vi "rad_Retrieve Image Wrapper.vi"(7 "Deployment Notifiers":T6, 8 "error in (no error)":errorcluster, 9 "AppImage Properties":T3, 10 "image file path":path, 11 "Target settings":T1={"Hostname"="", "Serial number"="", "Product name"="", "Product code"=0, "System status"="", "Credential type"=enum."None/Unlocked", "User added?"=FALSE, "Primary NIC"={"MAC address"="", "IP Address Request Mode"=2, "IP address"="", "Subnet mask"="", "Gateway"="", "DNS server"=""}} {"Primary NIC"."IP Address Request Mode" items=["Static"=1, "DHCP/Link-Local"=2, "Link-Local Only"=4, "DHCP Only"=8]}) -> (0 "error out":errorcluster, 3 "Canceled":bool)   [LabVIEW 2020]
uses:
  TypeDefs/rad_Deployment Progress Data Type.ctl
  TypeDefs/rad_Deployment Notifiers.ctl
  TypeDefs/rad_Deployment Status Data Type.ctl
  TypeDefs/rad_Application Image Properties.ctl
  TypeDefs/rad_FPGA Properties.ctl
  TypeDefs/rad_FPGA Flash Properties.ctl
  support/SubVIs/Target Information.ctl
  Targets/TypeDefs/rad_Target Network Settings.ctl
  <vilib>/nisyscfg/Software 1.2.ctl
  <vilib>/nisyscfg/Component Type.ctl
  <vilib>/nisyscfg/Create System Image (Folder).vi
  <vilib>/nisyscfg/Close (System).vi
  <vilib>/nisyscfg/nisyscfg.lvlib
panel:
  in  "Stop Checking for Events":bool
  out "Progress":T7 scale=0.0..100.0
  out "Status":string
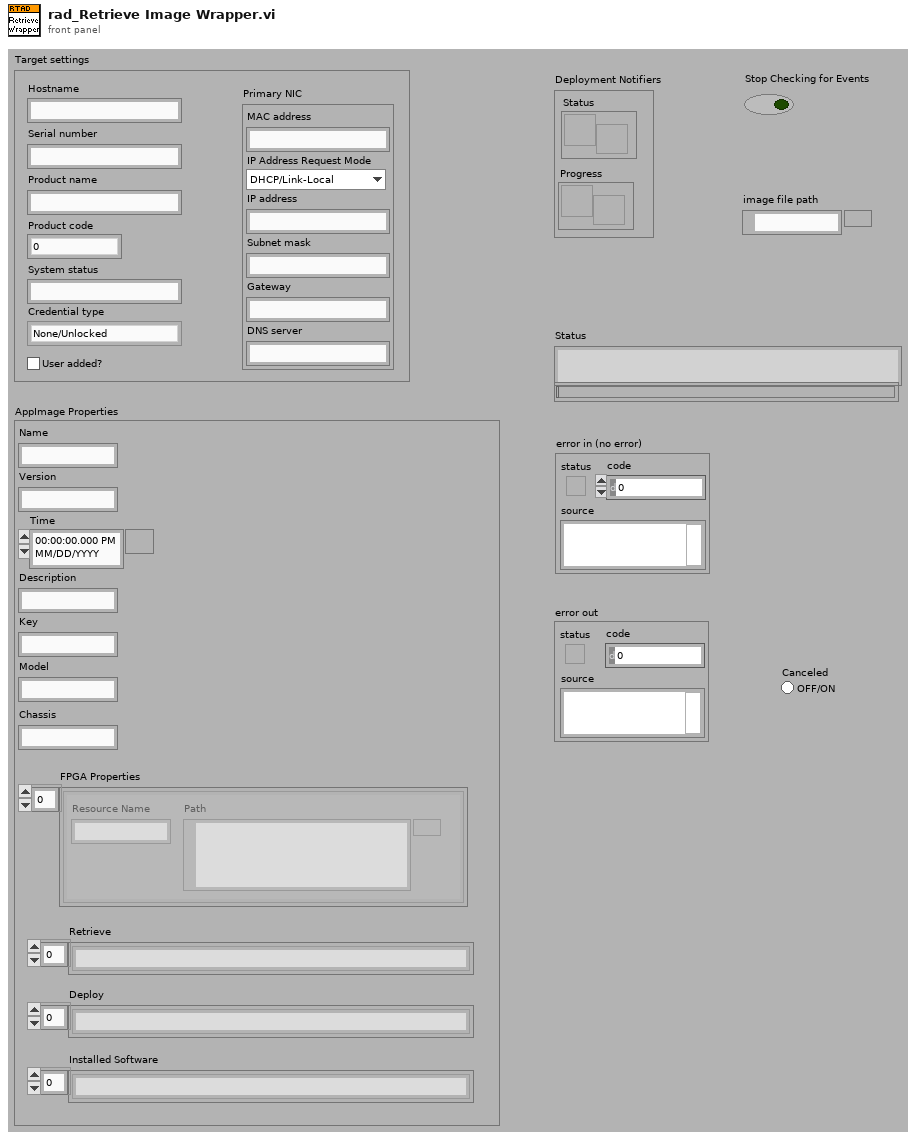
[diagram p1: front panel]
types:
  T1 = typedef "Target Information.ctl" = cluster{"Hostname":string, "Serial number":string, "Product name":string, "Product code":i32, "System status":string, "Credential type":enum16{"None/Unlocked", "FTP Password", "NIAuth Credentials"}, "User added?":bool, "Primary NIC":T2}
  T2 = typedef "rad_Target Network Settings.ctl" = cluster{"MAC address":string, "IP Address Request Mode":i32, "IP address":string, "Subnet mask":string, "Gateway":string, "DNS server":string}
  T3 = typedef "rad_Application Image Properties.ctl" = cluster{"Name":string, "Version":string, "Time":timestamp, "Description":string, "Key":string, "Chassis":string, "FPGA Properties":T4, "Model":string, "Retrieve":string[], "Deploy":string[], "Installed Software":string[]}
  T4 = typedef "rad_FPGA Properties.ctl" = T5[]
  T5 = typedef "rad_FPGA Flash Properties.ctl" = cluster{"Resource Name":string, "Path":path}
  T6 = typedef "rad_Deployment Notifiers.ctl" = cluster{"Status":refnum<notifier>, "Progress":refnum<notifier>}
  T7 = typedef "rad_Deployment Progress Data Type.ctl" = i8
  T8 = typedef "nisyscfg.lvlib/Software 1.2.ctl" = cluster{"title":string, "description":string, "ID":string, "version":string, "component type":T9}
  T9 = typedef "nisyscfg.lvlib/Component Type.ctl" = u32
  T10 = enum32{"state changed", "beginning restart", "getting file", "putting file", "creating directory", "deleting file", "deleting directory", "enumerating file system", "renaming file", "current component", "operation progress", "downloading file", "unpacking file", "running install script"}
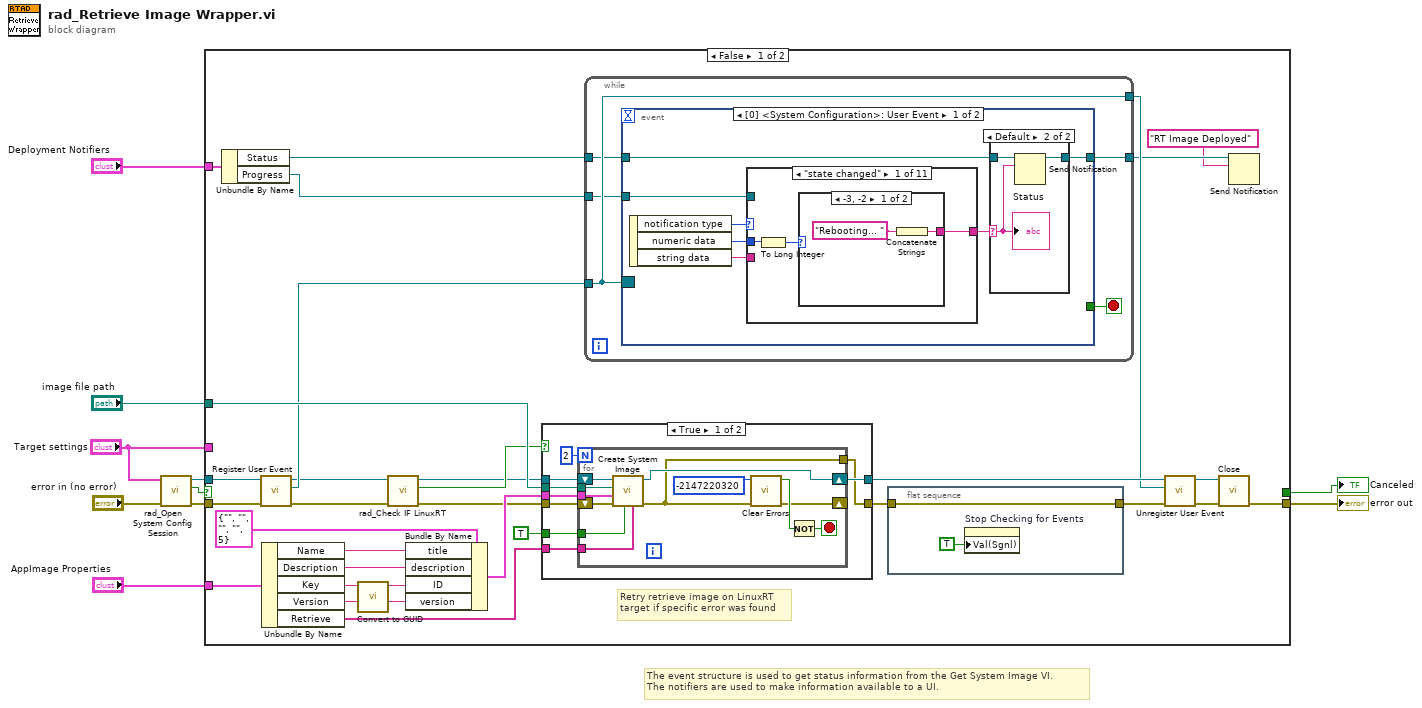
[diagram p0: block diagram]
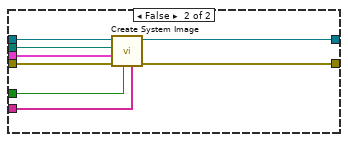
[diagram p2: hidden frame]
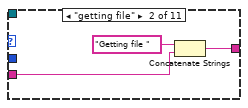
[diagram p5: hidden frame]
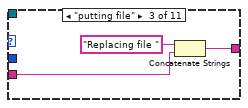
[diagram p6: hidden frame]
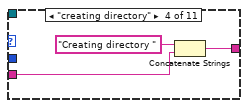
[diagram p7: hidden frame]
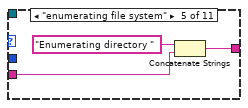
[diagram p8: hidden frame]
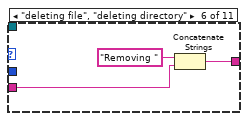
[diagram p9: hidden frame]
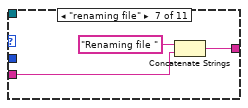
[diagram p10: hidden frame]
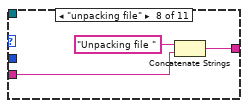
[diagram p11: hidden frame]
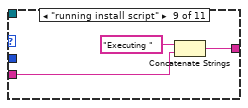
[diagram p12: hidden frame]
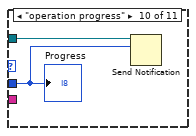
[diagram p13: hidden frame]
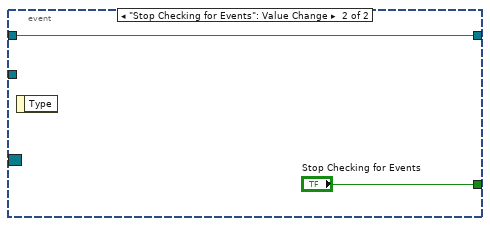
[diagram p15: hidden frame]
diagram:
  # "The event structure is used to get status information from the Get System Image VI. \nThe notifiers are used to make information available to a UI."
  n1 = call "rad_Open System Config Session.vi"("error in (no error)"="error in (no error)", "Target settings"="Target settings") -> ("error out"=w3:errorcluster, "Cancelled"=w2:bool, "Session out"=w4:refnum<k21>)  [unwired: 6 in, 1 out]
  n2 = case shown="False" w2 {
    selector: w2 -> [_ w122]
    tunnel: [w41 w123] -> w8
    tunnel: "image file path" -> [w40 _]
    tunnel: w4 -> [w39 _]
    tunnel: w3 -> [w38 w123]
    tunnel: "Deployment Notifiers" -> [w25 _]
    tunnel: "AppImage Properties" -> [w24 _]
    tunnel: [_ w122] -> w6
    tunnel: "Target settings" -> [_ _]
    frame False {
      # "Retry retrieve image on LinuxRT\ntarget if specific error was found"
      n3 = Unbundle By Name(w25) -> ("Status"=w27:refnum<notifier>, "Progress"=w26:refnum<notifier>)
      n4 = call <vilib>:"Register User Event.vi"("error in (no error)"=w38, "Session in"=w39) -> ("error out"=w14:errorcluster, "Event Registration out"=w37:refnum<event-registration>, "Session out"=w15:refnum<k21>)  [unwired: 7 in]
      n5 = Unbundle By Name(w24) -> ("Name"=w22:string, "Description"=w21:string, "Key"=w18:string, "Version"=w20:string, "Retrieve"=w16:string[])
      n6 = call "Convert to GUID.vi"("Key"=w18) -> ("GUID"=w17:string)  [unwired: 10 in]
      n7 = call "rad_Check IF LinuxRT.vi"("Error In"=w14, "System Session In"=w15) -> ("Error Out"=w11:errorcluster, "Target is LinuxRT?"=w13:bool, "System Session Out"=w12:refnum<k21>)  [unwired: 5 in, 2 out]
      n8 = Bundle By Name(cluster=T8 {"title"="", "description"="", "ID"="", "version"="", "component type"=5} ("image metadata"), "title"=w22, "description"=w21, "ID"=w17, "version"=w20) -> (w19:T8)
      n9 = case shown="True" w13 {
        tunnel: w40 -> [w50 w70]
        tunnel: w12 -> [w49 w69]
        tunnel: w11 -> [w48 w68]
        tunnel: [w47 w67] -> w34
        tunnel: [w42 w66] -> w32
        tunnel: TRUE ("overwrite (F)") -> [w46 w65]
        tunnel: w19 -> [w45 w64]
        tunnel: w16 -> [w44 w63]
        frame True {
          n10 = for {
            N: 2 -> [_]
            tunnel: w50 -> [w62]
            tunnel: w46 -> [w59]
            tunnel: w45 -> [w58]
            shift-right: [w54] -> w47
            shift-left: w49 -> [w61]
            shift-right: [w52] -> _
            shift-left: w48 -> [w60]
            tunnel: w44 -> [w57]
            tunnel: [w53] -> w42
            stop <- w56 stop-if-true
            n11 = call-poly <vilib>:"Create System Image.vi"("File and Directory Blacklist"=w57, "Overwrite (F)"=w59, "error in (no error)"=w60, "Image Metadata in"=w58, "Destination Folder"=w62, "Session in"=w61) -> ("error out"=w53:errorcluster, "Session out"=w54:refnum<k21>)  [unwired: 3 in, 1 out]
            n12 = call <vilib>:"Clear Errors.vi"("error in (no error)"=w53, "specific error code to clear (0: all)"=-2147220320) -> ("error out"=w52:errorcluster, "specific error cleared?"=w55:bool)  [unwired: 4 in]
            n13 = Not(x=w55) -> (.not. x?=w56:bool)
          }
        }
        frame False {
          n14 = call-poly <vilib>:"Create System Image.vi"("File and Directory Blacklist"=w63, "Overwrite (F)"=w65, "error in (no error)"=w68, "Image Metadata in"=w64, "Destination Folder"=w70, "Session in"=w69) -> ("error out"=w66:errorcluster, "Session out"=w67:refnum<k21>)  [unwired: 3 in, 1 out]
        }
      }
      n15 = while {
        tunnel: w37 -> [w77]
        tunnel: [w77] -> w33
        tunnel: w27 -> [w75]
        tunnel: [w74] -> w30
        tunnel: w26 -> [w73]
        stop <- w76 stop-if-true
        n16 = event shown="[0] <System Configuration>: User Event" {
          selector: w77 -> [_ _]
          dyn-events: _ -> [_ _]
          timeout: _ -> [_ _]
          tunnel: [_ "Stop Checking for Events"] -> w76
          tunnel: w75 -> [w80 w120]
          tunnel: [w79 w120] -> w74
          tunnel: w73 -> [w78 _]
          event User Event {
            n17 = event-data() -> ("notification type"=w84:T10, "numeric data"=w82:u32, "string data"=w83:string)  [unwired: 1 in]
            n18 = case shown="\"state changed\"" w84 {
              tunnel: [w89 w94 w97 w100 w103 w106 w109 w112 w115 _ _] -> w81
              tunnel: w83 -> [_ w95 w98 w101 w104 w107 w110 w113 w116 _ _]
              tunnel: w82 -> [w91 _ _ _ _ _ _ _ _ w118 _]
              tunnel: w78 -> [_ _ _ _ _ _ _ _ _ w119 _]
              frame "state changed" {
                n19 = To Long Integer(number=w91) -> (32bit integer=w90:i32)
                n20 = case shown="-3, -2" w90 {
                  tunnel: [w92 _] -> w89
                  frame -3, -2 {
                    n21 = Concatenate Strings("Rebooting... ") -> (w92:string)
                  }
                  frame Default {
                  }
                }
              }
              frame "getting file" {
                n22 = Concatenate Strings("Getting file " ("Status"), w95) -> (w94:string)
              }
              frame "putting file" {
                n23 = Concatenate Strings("Replacing file " ("Status"), w98) -> (w97:string)
              }
              frame "creating directory" {
                n24 = Concatenate Strings("Creating directory " ("Status"), w101) -> (w100:string)
              }
              frame "enumerating file system" {
                n25 = Concatenate Strings("Enumerating directory " ("Status"), w104) -> (w103:string)
              }
              frame "deleting file", "deleting directory" {
                n26 = Concatenate Strings("Removing " ("Status"), w107) -> (w106:string)
              }
              frame "renaming file" {
                n27 = Concatenate Strings("Renaming file " ("Status"), w110) -> (w109:string)
              }
              frame "unpacking file" {
                n28 = Concatenate Strings("Unpacking file " ("Status"), w113) -> (w112:string)
              }
              frame "running install script" {
                n29 = Concatenate Strings("Executing " ("Status"), w116) -> (w115:string)
              }
              frame "operation progress" {
                n30 = Send Notification(notification=w118, notifier=w119) -> ()  [unwired: 1 in, 2 out]
                "Progress" <- w118
              }
              frame Default {
              }
            }
            n31 = case shown="Default" w81 {
              selector: w81 -> [_ w87]
              tunnel: w80 -> [w85 w88]
              tunnel: [w85 w86] -> w79
              frame "" {
              }
              frame Default {
                n32 = Send Notification(notification=w87, notifier=w88) -> (notifier out=w86:refnum<notifier>)  [unwired: 1 in, 1 out]
                "Status" <- w87
              }
            }
          }
          event "Stop Checking for Events": Value Change {
            n33 = event-data() -> ()  [unwired: 1 in, 1 out]
          }
        }
      }
      n34 = flat-sequence {
        tunnel: w32 -> [w72]
        tunnel: [w72] -> w31
        frame #0 {
          n35 = property on="Stop Checking for Events" class="Bool (strict)"("Val(Sgnl)"=TRUE ("Stop Checking for Events")) -> ()  [unwired: 2 in, 2 out]
        }
      }
      n36 = call <vilib>:"Unregister User Event.vi"("error in (no error)"=w31, "Event Registration in"=w33, "Session in"=w34) -> ("error out"=w35:errorcluster, "Session out"=w36:refnum<k21>)  [unwired: 7 in]
      n37 = call-poly <vilib>:"Close.vi"("error in (no error)"=w35, "Session in"=w36) -> ("error out"=w41:errorcluster)  [unwired: 9 in]
      n38 = Send Notification(notification="RT Image Deployed", notifier=w30) -> ()  [unwired: 1 in, 2 out]
    }
    frame True {
    }
  }
  "error out" <- w8
  "Canceled" <- w6
